vi "OSICS_Read_MAV_GPIB.vi"(8 "error in":errorcluster, 11 "VISA IN":refnum<visa-resource-name>) -> (0 "error out":errorcluster, 2 "Message":string, 3 "VISA OUT":refnum<visa-resource-name>)   [LabVIEW 2014, in "OSICS_LIB.lvlib"]
doc: "This Vi reads a Message Available (MAV) in the buffer.\nGPIB only."
uses:
  OSICS_LIB.lvlib
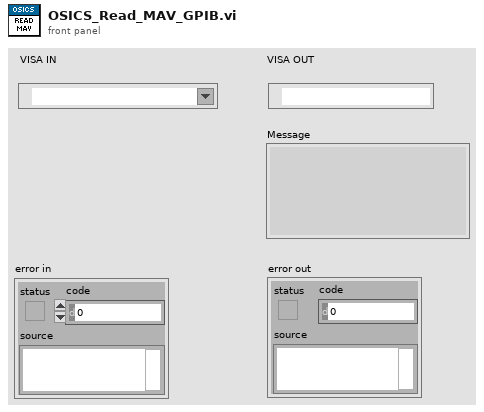
[diagram p1: front panel]
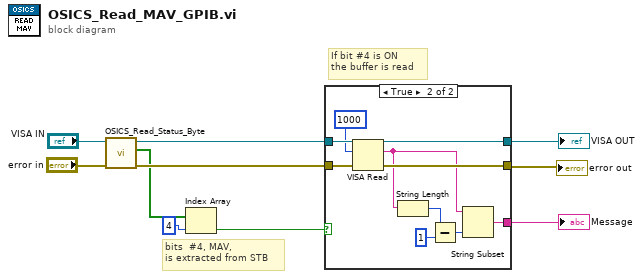
[diagram p0: block diagram]
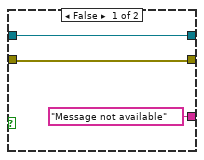
[diagram p2: hidden frame]
diagram:
  # "If bit #4 is ON\nthe buffer is read"
  # "bits  #4, MAV,\nis extracted from STB"
  n1 = call "OSICS_Read_Status_Byte.vi"("error in"="error in", "VISA IN"="VISA IN") -> ("error out"=w7:errorcluster, "SBR"=w2:bool[], "VISA OUT"=w8:refnum<visa-resource-name>)  [unwired: 7 in]
  n2 = Index Array(array=w2, index=4) -> (element=w4:bool)
  n3 = case shown="True" w4 {
    tunnel: w8 -> [w13 w23]
    tunnel: w7 -> [w12 w22]
    tunnel: [w12 w20] -> w6
    tunnel: [w13 w14] -> w5
    tunnel: ["Message not available" ("read buffer") w15] -> w3
    frame False {
    }
    frame True {
      n4 = VISA Read(VISA resource name=w23, byte count=u32 1000, error in (no error)=w22) -> (VISA resource name out=w14:refnum<visa-resource-name>, read buffer=w16:string, error out=w20:errorcluster)  [unwired: 1 out]
      n5 = String Length(string=w16) -> (length=w18:i32)
      n6 = Subtract(x=w18, y=1) -> (x-y=w17:i32)
      n7 = String Subset(string=w16, length (rest)=w17) -> (substring=w15:string)  [unwired: 1 out]
    }
  }
  "error out" <- w6
  "VISA OUT" <- w5
  "Message" <- w3
